vi "Command builder.vi"(8 "error in":errorcluster, 11 "Config path":path=path "C:/Users/ken_X/Documents/LabVIEW projects/Project-B2/settings/config.xls") -> (0 "error out":errorcluster, 2 "Commands":string[][](array[string]))   [LabVIEW 2021]
uses:
  <vilib>/Utility/file.llb/Read Delimited Spreadsheet (string).vi
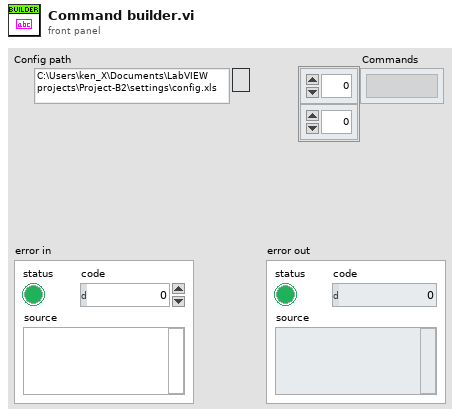
[diagram p1: front panel]
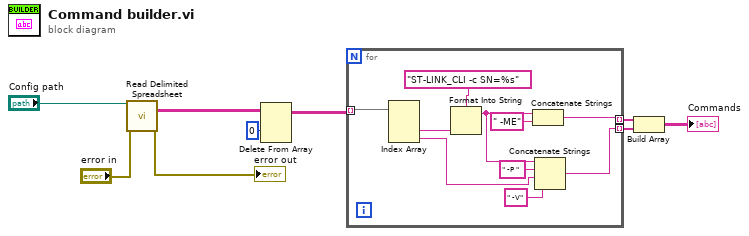
[diagram p0: block diagram]
diagram:
  n1 = call-poly <vilib>:"Read Delimited Spreadsheet.vi"("file path (dialog if empty)"="Config path", "error in (no error)"="error in") -> ("all rows"=w8:string[][], "error out"=→"error out":errorcluster)  [unwired: 8 in, 4 out]
  n2 = Delete From Array(array=w8, index (row)=0) -> (array with subset deleted=w7:string[][])  [unwired: 2 in, 1 out]
  n3 = for {
    tunnel: w7 -> [w19] mode=indexing
    tunnel: [w11] -> w2 mode=indexing
    tunnel: [w10] -> w3 mode=indexing
    n4 = Index Array(array=w19) -> (element #2=w17:string, element #3=w13:string)  [unwired: 3 in, 1 out]
    n5 = Format Into String(format string="ST-LINK_CLI -c SN=%s", w17) -> (resulting string=w15:string)  [unwired: 2 in, 1 out]
    n6 = Concatenate Strings(w15, " -ME" ("string")) -> (w10:string)
    n7 = Concatenate Strings(w15, " -P " ("string"), w13, " -V" ("string")) -> (w11:string)
  }
  n8 = Build Array(w3, w2) -> (→"Commands":string[][])
